vi "Main Page.vi"(8 "error in (no error)":errorcluster, 11 "Node Ptr":T2 format="%.0x") -> (0 "error out":errorcluster)   [LabVIEW 2019, in "TimingDRV System Explorer.lvlib"]
uses:
  TimingDRV System Explorer.lvlib
  <vilib>/NI VeriStand/Custom Device API/Custom Device Item Ref.ctl
  TypeDefs/Generator Types.ctl
  Engine/Parent Classes/Process/Process.lvclass
  Engine/Processes/Sine Process/Sine Process.lvclass
  C:/Users/XEnderMD/Desktop/CD Project Tools/Source/Engine/Parent Classes/Process/Process.lvclass
  Engine/Processes/Random Process/Random Process.lvclass
  <vilib>/NI VeriStand/Custom Device API/Set Item Property (String).vi
  <vilib>/NI VeriStand/Custom Device API/Custom Device API.lvlib
panel:
  out "Replaced ?":bool
  in  "Generator":T1
  in  "Header":cluster{"Section Name":string}={"Section Name"="Custom Device Item Settings"}
  in  "Description":string
  in  "Name":string
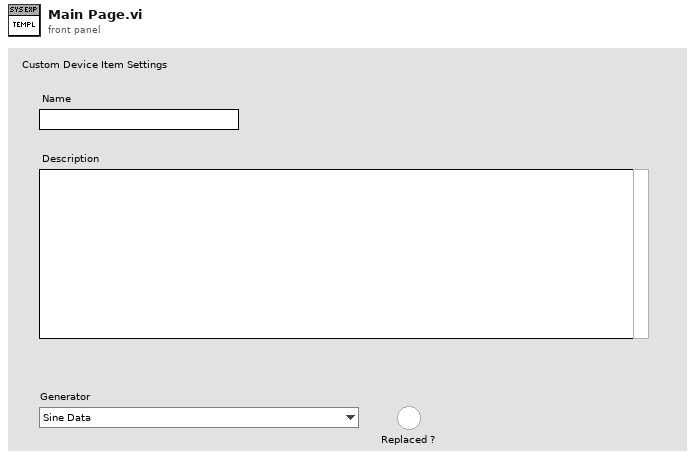
[diagram p1: front panel]
types:
  T1 = typedef "TimingDRV System Explorer.lvlib/Generator Types.ctl" = enum16{"Sine Data", "Random Data"}
  T2 = typedef "Custom Device API.lvlib/Custom Device Item Ref.ctl" = u64
  T3 = typedef "Custom Device API.lvlib/Custom Device Item Info.ctl" = cluster{"Name":string, "Is Channel":bool, "GUID":string, "Is Waveform":bool}
  T4 = typedef "Custom Device API.lvlib/Custom Device Commands.ctl" = enum16{"Default", "Item renamed", "Shutdown", "Dynamic button pressed"}
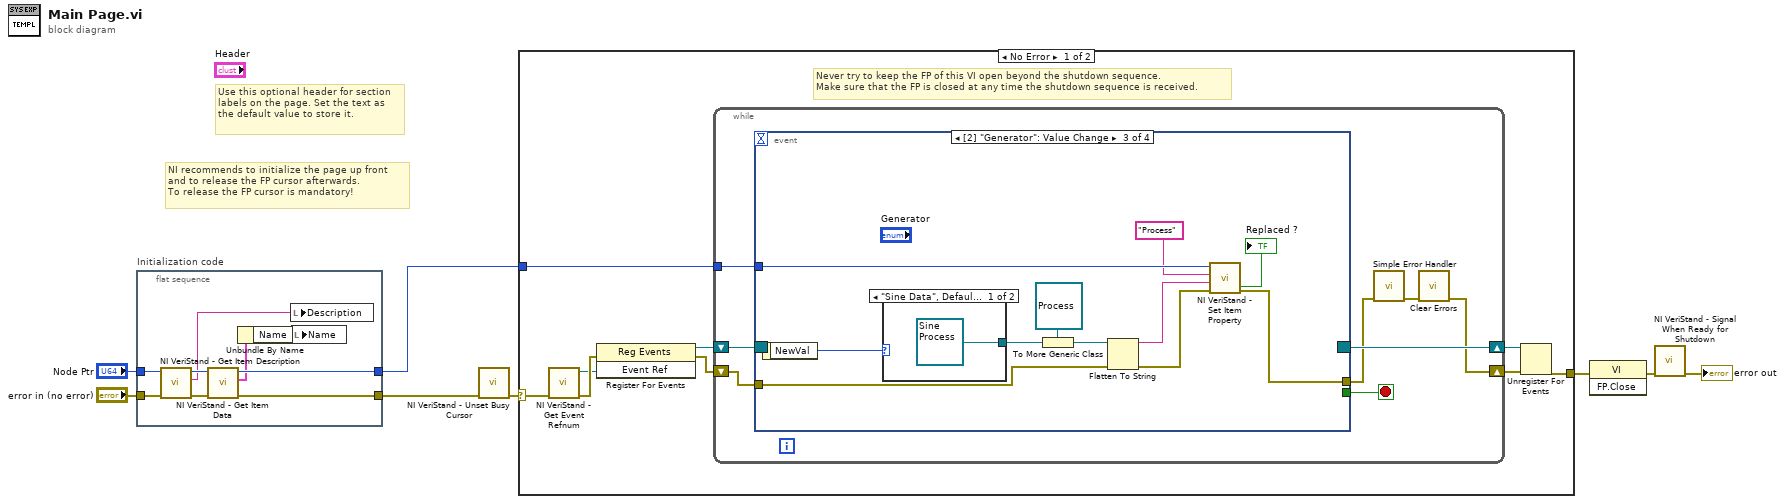
[diagram p0: block diagram]
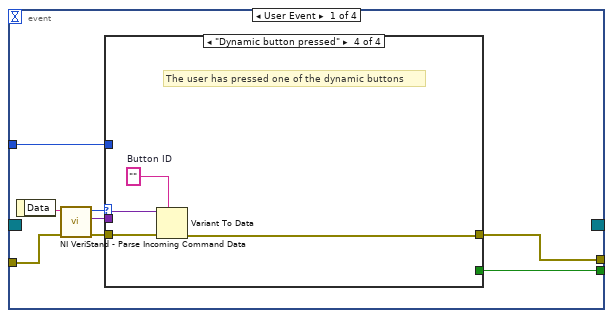
[diagram p2: hidden frame]
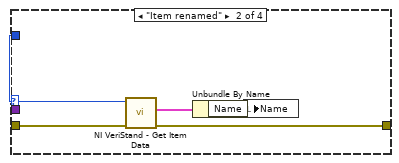
[diagram p4: hidden frame]
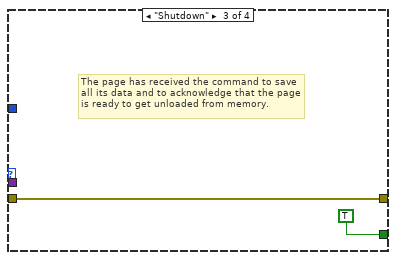
[diagram p5: hidden frame]
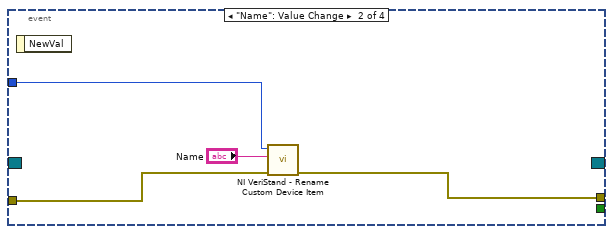
[diagram p6: hidden frame]
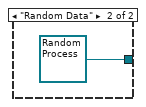
[diagram p7: hidden frame]
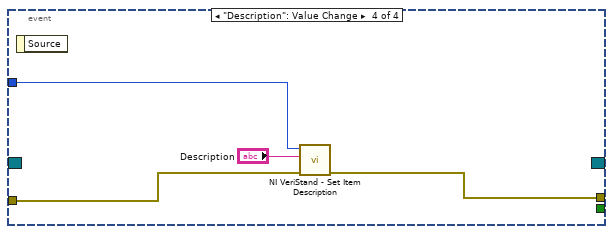
[diagram p8: hidden frame]
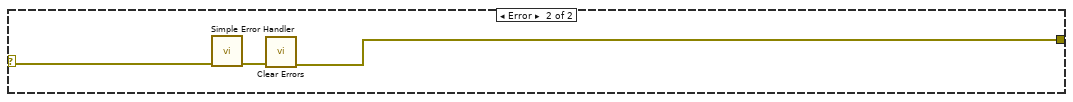
[diagram p9: hidden frame]
diagram:
  # "Use this optional header for section labels on the page. Set the text as the default value to store it."
  # "NI recommends to initialize the page up front\nand to release the FP cursor afterwards.\nTo release the FP cursor is mandatory!"
  n1 = flat-sequence "Initialization code" {
    tunnel: "error in (no error)" -> [w15]
    tunnel: "Node Ptr" -> [w14]
    tunnel: [w9] -> w1
    tunnel: [w17] -> w2
    frame #0 {
      n2 = call <vilib>:"NI VeriStand - Get Item Description.vi"("error in (no error)"=w15, "Item Ref in"=w14) -> ("error out"=w12:errorcluster, "Description"=w13:string, "Item Ref out"=w16:T2)  [unwired: 7 out]
      n3 = call <vilib>:"NI VeriStand - Get Item Data.vi"("error in (no error)"=w12, "Item Ref in"=w16) -> ("error out"=w9:errorcluster, "Item Info"=w11:T3, "Item Ref out"=w17:T2)  [unwired: 7 out]
      n4 = Unbundle By Name(w11) -> ("Name"=w10:string)
      n5 = local write "Description"(w13) -> ()
      n6 = local write "Name"(w10) -> ()
    }
  }
  n7 = call <vilib>:"NI VeriStand - Unset Busy Cursor.vi"("error in (no error)"=w1) -> ("error out"=w4:errorcluster)  [unwired: 10 out]
  n8 = case shown="No Error" w4 {
    selector: w4 -> [w19 w78]
    tunnel: [w23 w76] -> w8
    tunnel: w2 -> [w20 _]
    frame No Error {
      # "Never try to keep the FP of this VI open beyond the shutdown sequence.\nMake sure that the FP is closed at any time the shutdown sequence is received."
      n9 = call <vilib>:"NI VeriStand - Get Event Refnum.vi"("error in (no error)"=w19) -> ("error out"=w26:errorcluster, "Event Ref"=w22:refnum<user-event>)  [unwired: 9 out]
      n10 = register-events(error in=w26, w22) -> (reference out=w21:refnum<event-registration>, error out=w18:errorcluster)  [unwired: 1 in]
      n11 = while {
        tunnel: w20 -> [w30]
        shift-right: [w27] -> w24
        shift-left: w18 -> [w33]
        shift-right: [w34] -> w25
        shift-left: w21 -> [w32]
        stop <- w31 stop-if-true
        n12 = event shown="[2] \"Generator\": Value Change" {
          selector: w32 -> [_ _ _ _]
          dyn-events: [_ _ _ _] -> w34
          timeout: _ -> [_ _ _ _]
          tunnel: w33 -> [w42 w58 w63 w74]
          tunnel: [w38 _ _ _] -> w31
          tunnel: [w37 w57 w65 w73] -> w29
          tunnel: w30 -> [w36 w56 w68 w75]
          event User Event {
            n13 = event-data() -> ("Data"=w41:string)  [unwired: 1 out]
            n14 = call <vilib>:"NI VeriStand - Parse Incoming Command Data.vi"("error in (no error)"=w42, "Incoming data"=w41) -> ("error out"=w40:errorcluster, "Outgoing data"=w35:variant, "Action"=w39:T4)  [unwired: 7 out]
            n15 = case shown="\"Dynamic button pressed\"" w39 {
              tunnel: w40 -> [w43 w48 w49 w54]
              tunnel: [_ _ TRUE _] -> w38
              tunnel: [w43 w45 w49 w51] -> w37
              tunnel: w36 -> [_ w47 _ _]
              tunnel: w35 -> [_ _ _ w53]
              frame "Default", Default {
              }
              frame "Item renamed" {
                n16 = call <vilib>:"NI VeriStand - Get Item Data.vi"("error in (no error)"=w48, "Item Ref in"=w47) -> ("error out"=w45:errorcluster, "Item Info"=w46:T3)  [unwired: 8 out]
                n17 = Unbundle By Name(w46) -> ("Name"=w44:string)
                n18 = local write "Name"(w44) -> ()
              }
              frame "Shutdown" {
                # "The page has received the command to save all its data and to acknowledge that the page is ready to get unloaded from memory."
              }
              frame "Dynamic button pressed" {
                w52 = ""  # Button ID
                # "The user has pressed one of the dynamic buttons"
                n19 = Variant To Data(error in=w54, type=w52, Variant=w53) -> (error out=w51:errorcluster)  [unwired: 1 out]
              }
            }
          }
          event "Name": Value Change {
            n20 = event-data() -> ()  [unwired: 2 out]
            n21 = call <vilib>:"NI VeriStand - Rename Custom Device Item.vi"("error in (no error)"=w58, "New Name"="Name", "Item Ref in"=w56) -> ("error out"=w57:errorcluster)  [unwired: 1 in, 7 out]
          }
          event Value Change {
            n22 = event-data() -> ("NewVal"=w69:T1)  [unwired: 1 out]
            n23 = case shown="\"Sine Data\", Default" w69 {
              tunnel: [refnum<class "Sine Process.lvclass"> refnum ("TelemetryAsync Engine.lvlib:Sine Process.lvclass") refnum<class "Random Process.lvclass"> refnum ("TelemetryAsync Engine.lvlib:Random Process.lvclass")] -> w67
              frame "Sine Data", Default {
              }
              frame "Random Data" {
              }
            }
            n24 = To More Generic Class(target class=refnum<class "Process.lvclass"> refnum ("TelemetryAsync Engine.lvlib:Process.lvclass"), reference=w67) -> (generic class reference=w64:refnum<class "Process.lvclass">)
            n25 = Flatten To String(anything=w64, error in (no error)=w63) -> (data string=w61:string, error out=w62:errorcluster)  [unwired: 2 in, 1 out]
            n26 = call-poly <vilib>:"NI VeriStand - Set Item Property.vi"("error in (no error)"=w62, "Value"=w61, "Property Name"="Process", "Item Ref in"=w68) -> ("error out"=w65:errorcluster, "Replaced"=→"Replaced ?":bool)  [unwired: 5 in, 1 out]
          }
          event "Description": Value Change {
            n27 = event-data() -> ()  [unwired: 2 out]
            n28 = call <vilib>:"NI VeriStand - Set Item Description.vi"("error in (no error)"=w74, "Description"="Description", "Item Ref in"=w75) -> ("error out"=w73:errorcluster)  [unwired: 8 out]
          }
        }
        n29 = call <vilib>:"Simple Error Handler.vi"("error in (no error)"=w29) -> ("error out"=w28:errorcluster)  [unwired: 1 in, 7 out]
        n30 = call <vilib>:"Clear Errors.vi"("error in (no error)"=w28) -> ("error out"=w27:errorcluster)  [unwired: 1 in, 5 out]
      }
      n31 = Unregister For Events(event registration refnum=w25, error in=w24) -> (error out=w23:errorcluster)
    }
    frame Error {
      n32 = call <vilib>:"Simple Error Handler.vi"("error in (no error)"=w78) -> ("error out"=w77:errorcluster)  [unwired: 1 in, 7 out]
      n33 = call <vilib>:"Clear Errors.vi"("error in (no error)"=w77) -> ("error out"=w76:errorcluster)  [unwired: 1 in, 5 out]
    }
  }
  n34 = invoke class="VI" method="FP.Close"(error in=w8) -> (error out=w7:errorcluster)  [unwired: 2 in, 2 out]
  n35 = call <vilib>:"NI VeriStand - Signal When Ready for Shutdown.vi"("error in (no error)"=w7) -> ("error out"=→"error out":errorcluster)  [unwired: 10 out]
